vi "Processing.vi"() -> ()   [LabVIEW 2016]
uses:
  <vilib>/Analysis/baseanly.llb/Mean (DBL).vi
  <vilib>/Analysis/NI_AALBase.lvlib
panel:
  out "mean":dbl[](array[numeric]) caption="Média" format="%.3g"
  out "max":dbl[](array[numeric]) caption="Máximo" format="%.3g"
  out "graph":waveform(dbl)[](graph)
  in  "file":path caption="Arquivo"
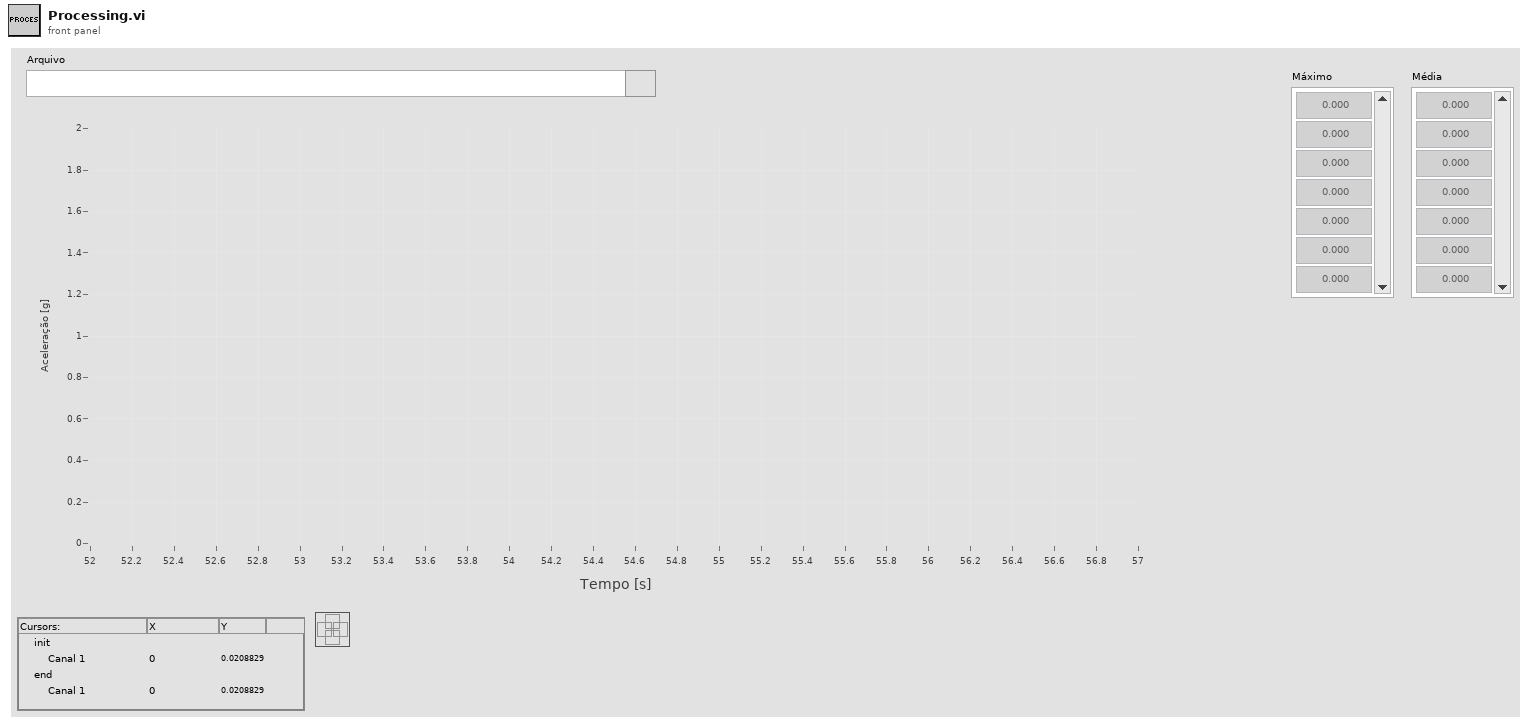
[diagram p1: front panel]
types:
  T1 = cluster{"seconds since 1Jan1904":timestamp, dbl[]}
  T2 = cluster{"seconds since 1Jan1904":timestamp, dbl[]}[]
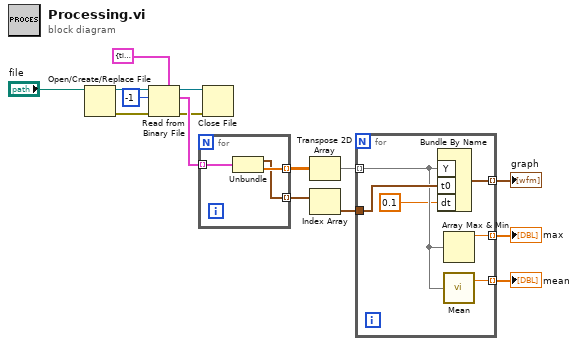
[diagram p0: block diagram]
diagram:
  n1 = Open/Create/Replace File(file path (use dialog)="file") -> (refnum out=w14:refnum<file>, error out=w13:errorcluster)  [unwired: 5 in, 1 out]
  n2 = Read from Binary File(5:T1 {"seconds since 1Jan1904"=timestamp(0 s since 1904-01-01), []} ("output cluster"), 8:w13, 10:-1 ("count (1)"), 11:w14) -> (0:w8:errorcluster, 2:w10:T2, 3:w7:refnum<file>)  [unwired: 2 in, 1 out]
  n3 = for {
    tunnel: w10 -> [w18] mode=indexing
    tunnel: [w17] -> w9 mode=indexing
    tunnel: [w16] -> w6 mode=indexing
    n4 = Unbundle(w18) -> ("seconds since 1Jan1904"=w16:timestamp, w17:dbl[])
  }
  n5 = Close File(refnum=w7, error in=w8) -> ()  [unwired: 2 out]
  n6 = Transpose 2D Array(2D array=w9) -> (transposed array=w5:dbl[][])
  n7 = Index Array(array=w6) -> (element=w4:timestamp)  [unwired: 1 in]
  n8 = for {
    tunnel: w5 -> [w20] mode=indexing
    tunnel: w4 -> [w24]
    tunnel: [w23] -> w3 mode=indexing
    tunnel: [w22] -> w1 mode=indexing
    tunnel: [w21] -> w2 mode=indexing
    n9 = Bundle By Name("Y"=w20, "t0"=w24, "dt"=0.1) -> (w23:waveform(dbl))  [unwired: 1 in]
    n10 = Array Max & Min(array=w20) -> (max value=w22:dbl)  [unwired: 3 out]
    n11 = call-poly <vilib>:"Mean.vi"("X"=w20) -> ("mean"=w21:dbl)  [unwired: 1 out]
  }
  "graph" <- w3
  "max" <- w1
  "mean" <- w2
